vi "FG Camera HB.vi"(1 "FG Action (Read)":T1, 2 "Camera HB in":bool) -> (0 "Camera HB out":bool)   [LabVIEW 2009]
uses:
  Actions for FG's.ctl
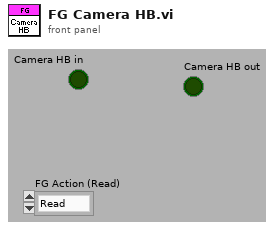
[diagram p1: front panel]
types:
  T1 = typedef "Actions for FG's.ctl" = enum16{"Read", "Write"}
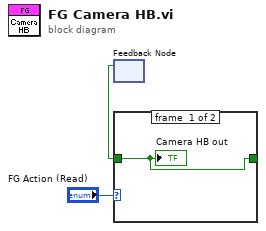
[diagram p0: block diagram]
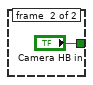
[diagram p2: hidden frame]
diagram:
  n1 = feedback #1() -> (w1:bool)  [unwired: 1 in]
  n2 = case shown="\"Read\", Default" "FG Action (Read)" {
    tunnel: w1 -> [w4 _]
    tunnel: [w4 "Camera HB in"] -> w2
    frame #0 {
      "Camera HB out" <- w4
    }
    frame #1 {
    }
  }
